vi "Exp header-Save cal header info.vi"(8 "error in (no error)":errorcluster, 11 "Experiment folder path":path) -> (0 "error out":errorcluster)   [LabVIEW 2013]
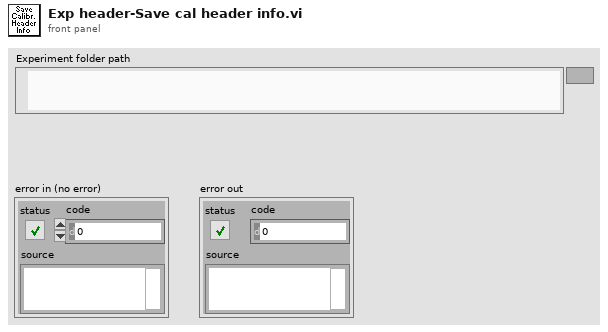
[diagram p1: front panel]
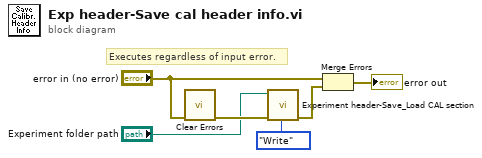
[diagram p0: block diagram]
diagram:
  # "Executes regardless of input error."
  n1 = call <vilib>:"Clear Errors.vi"("error in (no error)"="error in (no error)") -> ("error out"=w2:errorcluster)  [unwired: 6 in]
  n2 = call "Experiment header-Save_Load CAL section.vi"("error in (no error)"=w2, "Function"=enum16{"Write", "Read"}."Write", "Experiment folder path"="Experiment folder path") -> ("error out"=w3:errorcluster)  [unwired: 7 in, 1 out]
  n3 = Merge Errors("error in (no error)", w3) -> (→"error out":errorcluster)
